vi "DSP_SetStatus.vi"(2 "error in (no error)":errorcluster, 3 "Status":u32, 4 "Board Handle":u64) -> (0 "error out":errorcluster, 1 "Board Handle Out":u64)   [LabVIEW 2009]
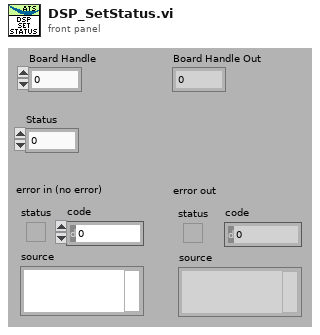
[diagram p1: front panel]
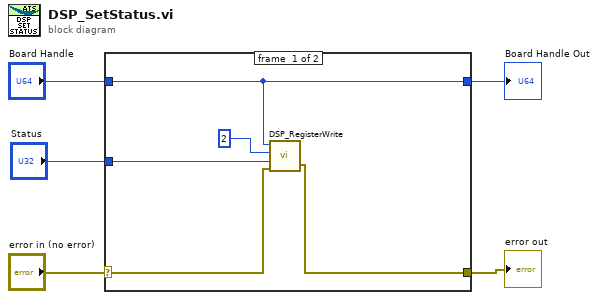
[diagram p0: block diagram]
diagram:
  n1 = case shown="No Error" "error in (no error)" {
    selector: "error in (no error)" -> [w9 w12]
    tunnel: [w8 w12] -> w4
    tunnel: [w10 w11] -> w3
    tunnel: "Board Handle" -> [w10 w11]
    tunnel: "Status" -> [w6 _]
    frame #0 {
      n2 = call "DSP_RegisterWrite.vi"("error in (no error)"=w9, "Value"=w6, "Offset"=u32 2, "Board Handle"=w10) -> ("error out"=w8:errorcluster)  [unwired: 1 out]
    }
    frame #1 {
    }
  }
  "Board Handle Out" <- w3
  "error out" <- w4
